vi "configgap.vi"(1 "zhomespeed":dbl, 2 "gap":dbl, 3 "gapspeed":dbl, 4 "连接ID":refnum<k5>) -> (0 "连接ID输出":refnum<k5>)   [LabVIEW 2017]
uses:
  <vilib>/LVH/i3 JSON/JSON Generation/Add Object Parameter Files/Add Object Parameter - Numeric.vi
  <vilib>/LVH/i3 JSON/i3-json.lvlib
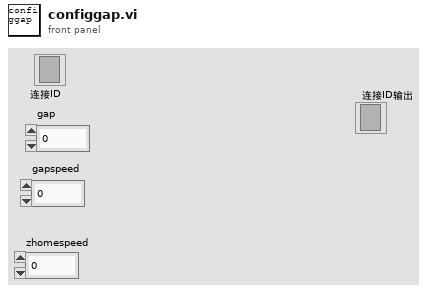
[diagram p1: front panel]
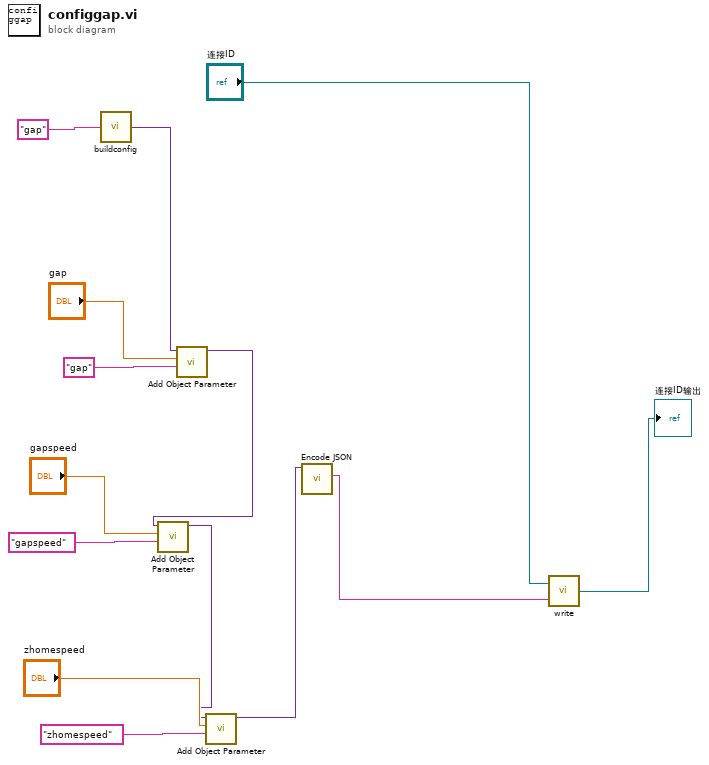
[diagram p0: block diagram]
diagram:
  n1 = call "buildconfig.vi"("String"="gap") -> ("JSON Tree out (JSON Object)"=w11:variant)
  n2 = call-poly <vilib>:"Add Object Parameter.vi"("Name"="gap", "Numeric"="gap", "JSON Tree in (JSON Object)"=w11) -> ("JSON Tree out (JSON Object)"=w5:variant)  [unwired: 7 in, 1 out]
  n3 = call-poly <vilib>:"Add Object Parameter.vi"("Name"="gapspeed", "Numeric"="gapspeed", "JSON Tree in (JSON Object)"=w5) -> ("JSON Tree out (JSON Object)"=w2:variant)  [unwired: 7 in, 1 out]
  n4 = call-poly <vilib>:"Add Object Parameter.vi"("Name"="zhomespeed", "Numeric"="zhomespeed", "JSON Tree in (JSON Object)"=w2) -> ("JSON Tree out (JSON Object)"=w1:variant)  [unwired: 7 in, 1 out]
  n5 = call <vilib>:"Encode JSON.vi"("JSON Tree"=w1) -> ("String"=w9:string)  [unwired: 5 in, 1 out]
  n6 = call "write.vi"("数据输入"=w9, "连接ID"="连接ID") -> ("连接ID输出"=→"连接ID输出":refnum<k5>)
